vi "cancelCallbacks.vi"(8 "error in (no error)":errorcluster, 11 "MiddlewareSALThisComponent in":refnum<class "MiddlewareSALThisComponent.lvclass">) -> (0 "error out":errorcluster, 3 "MiddlewareSALThisComponent out":refnum<class "MiddlewareSALThisComponent.lvclass">)   [LabVIEW 2016, in "MiddlewareSALThisComponent.lvclass"]
uses:
  MiddlewareSALThisComponent.lvclass
  ts_sallv_FiberSpectrograph/SALLV_FiberSpectrograph.lvlib
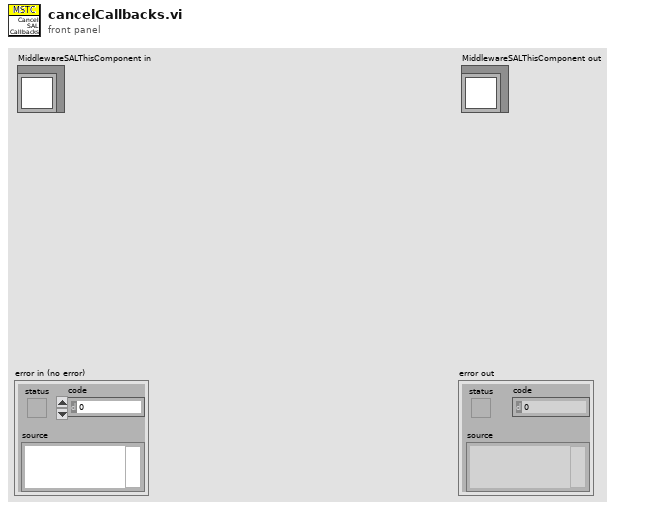
[diagram p1: front panel]
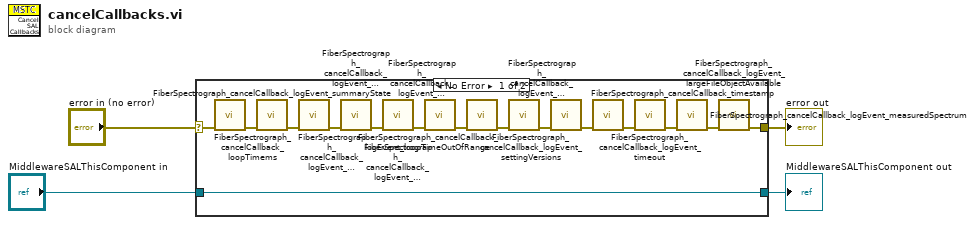
[diagram p0: block diagram]
diagram:
  n1 = case shown="No Error" "error in (no error)" {
    selector: "error in (no error)" -> [w5 w21]
    tunnel: [w16 w21] -> w3
    tunnel: [w19 w20] -> w1
    tunnel: "MiddlewareSALThisComponent in" -> [w19 w20]
    frame No Error {
      n2 = call "FiberSpectrograph_cancelCallback_loopTimems.vi"("error in (no error)"=w5) -> ("error out"=w6:errorcluster)  [unwired: 9 in, 1 out]
      n3 = call "FiberSpectrograph_cancelCallback_logEvent_summaryState.vi"("error in (no error)"=w6) -> ("error out"=w7:errorcluster)  [unwired: 9 in, 1 out]
      n4 = call "FiberSpectrograph_cancelCallback_logEvent_appliedSettingsMatchStart.vi"("error in (no error)"=w7) -> ("error out"=w8:errorcluster)  [unwired: 9 in, 1 out]
      n5 = call "FiberSpectrograph_cancelCallback_logEvent_detailedState.vi"("error in (no error)"=w8) -> ("error out"=w9:errorcluster)  [unwired: 9 in, 1 out]
      n6 = call "FiberSpectrograph_cancelCallback_logEvent_errorCode.vi"("error in (no error)"=w9) -> ("error out"=w10:errorcluster)  [unwired: 9 in, 1 out]
      n7 = call "FiberSpectrograph_cancelCallback_logEvent_heartbeat.vi"("error in (no error)"=w10) -> ("error out"=w11:errorcluster)  [unwired: 9 in, 1 out]
      n8 = call "FiberSpectrograph_cancelCallback_logEvent_loopTimeOutOfRange.vi"("error in (no error)"=w11) -> ("error out"=w12:errorcluster)  [unwired: 9 in, 1 out]
      n9 = call "FiberSpectrograph_cancelCallback_logEvent_rejectedCommand.vi"("error in (no error)"=w12) -> ("error out"=w13:errorcluster)  [unwired: 9 in, 1 out]
      n10 = call "FiberSpectrograph_cancelCallback_logEvent_settingVersions.vi"("error in (no error)"=w13) -> ("error out"=w14:errorcluster)  [unwired: 9 in, 1 out]
      n11 = call "FiberSpectrograph_cancelCallback_timestamp.vi"("error in (no error)"=w14) -> ("error out"=w15:errorcluster)  [unwired: 9 in, 1 out]
      n12 = call "FiberSpectrograph_cancelCallback_logEvent_timeout.vi"("error in (no error)"=w15) -> ("error out"=w18:errorcluster)  [unwired: 9 in, 1 out]
      n13 = call "FiberSpectrograph_cancelCallback_logEvent_measuredSpectrum.vi"("error in (no error)"=w18) -> ("error out"=w17:errorcluster)  [unwired: 9 in, 1 out]
      n14 = call "FiberSpectrograph_cancelCallback_logEvent_largeFileObjectAvailable.vi"("error in (no error)"=w17) -> ("error out"=w16:errorcluster)  [unwired: 9 in, 1 out]
    }
    frame Error {
    }
  }
  "error out" <- w3
  "MiddlewareSALThisComponent out" <- w1
